vi "Template RF Test Get Default Parameters.vi"(8 "error in (no error)":errorcluster, 11 "Template Tx Test in":refnum<class "Template RF Test.lvclass">) -> (0 "error out":errorcluster, 2 "Parameters":T1, 3 "Template Tx Test out":refnum<class "Template RF Test.lvclass">)   [LabVIEW 2015, in "niDTS Template.lvlib" / "Template RF Test.lvclass"]
uses:
  Template RF Test.lvclass
  Includes/Template RF Test INC Parameters.ctl
  Template RF Test.lvclass/Template RF Test.ctl
  niDTS Template.lvlib
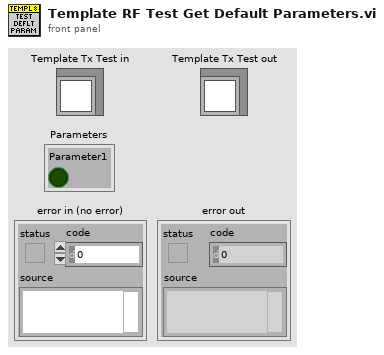
[diagram p1: front panel]
types:
  T1 = typedef "niDTS Template.lvlib/Template RF Test INC Parameters.ctl" = cluster{"Parameter1":bool}
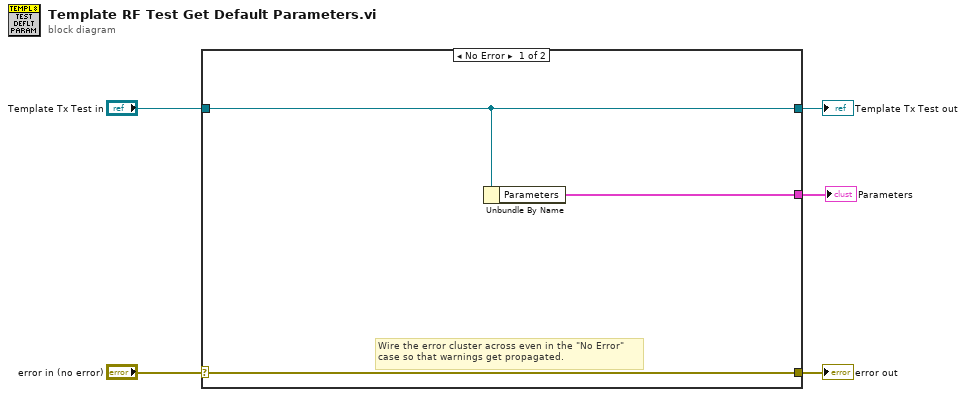
[diagram p0: block diagram]
diagram:
  n1 = case shown="No Error" "error in (no error)" {
    selector: "error in (no error)" -> [w8 w10]
    tunnel: [w8 w10] -> w4
    tunnel: [w7 w9] -> w2
    tunnel: "Template Tx Test in" -> [w7 w9]
    tunnel: [w6 _] -> w1
    frame No Error {
      # "Wire the error cluster across even in the \"No Error\"\ncase so that warnings get propagated."
      n2 = Unbundle By Name(w7) -> ("Parameters"=w6:T1)
    }
    frame Error {
    }
  }
  "error out" <- w4
  "Template Tx Test out" <- w2
  "Parameters" <- w1
